vi "aquisicao.vi"() -> ()   [LabVIEW 2018]
uses:
  <vilib>/DAQmx/read.llb/DAQmx Read (Analog 1D Wfm NChan NSamp).vi
  <vilib>/DAQmx/create/channels.llb/DAQmx Create Channel (AI-Voltage-Basic).vi
  <vilib>/DAQmx/configure/timing.llb/DAQmx Timing (Sample Clock).vi
  <vilib>/DAQmx/miscellaneous.llb/DAQmx Fill In Error Info.vi
panel:
  in  "Parar":bool caption="stop"
  out "Onda Gerada":waveform(dbl)[](graph)
  # "Validação da Onda Gerada"
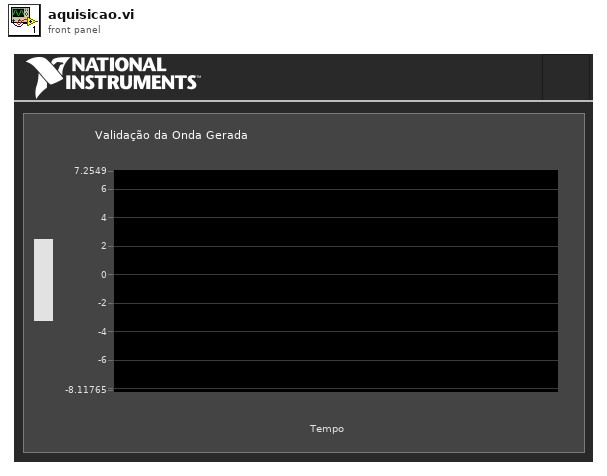
[diagram p1: front panel]
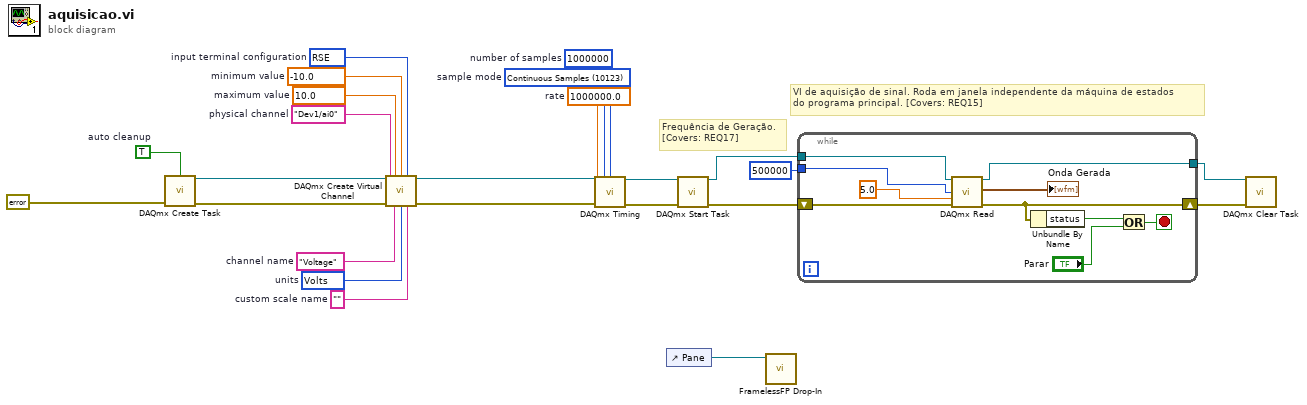
[diagram p0: block diagram]
diagram:
  w17 = 10123 items=["Finite Samples"=10178, "Continuous Samples"=10123, "Hardware Timed Single Point"=12522]  # sample mode
  w16 = 1000000  # number of samples
  w15 = 1000000.0  # rate
  w13 = 10083 items=["default"=-1, "RSE"=10083, "NRSE"=10078, "Differential"=10106, "Pseudodifferential"=12529]  # input terminal configuration
  w12 = 10348 items=["Volts"=10348, "From Custom Scale"=10065]  # units
  w11 = "Voltage"  # channel name
  w9 = ""  # custom scale name
  w8 = -10.0  # minimum value
  w7 = 10.0  # maximum value
  w6 = "Dev1/ai0"  # physical channel
  w4 = TRUE  # auto cleanup
  # "Frequência de Geração.\n[Covers: REQ17]"
  # "VI de aquisição de sinal. Roda em janela independente da máquina de estados\ndo programa principal. [Covers: REQ15]"
  n1 = call <vilib>:"DAQmx Create Task.vi"("auto cleanup"=w4, "error in"=errorcluster {"status"=FALSE, "code"=0, "source"=""}) -> ("task out"=w5:refnum<k21>, "error out"=w3:errorcluster)  [unwired: 12 in]
  n2 = call-poly <vilib>:"DAQmx Create Virtual Channel.vi"("task in"=w5, "maximum value"=w7, "minimum value"=w8, "input terminal configuration"=w13, "physical channels"=w6, "name to assign"=w11, "units"=w12, "error in"=w3, "custom scale name"=w9) -> ("task out"=w14:refnum<k21>, "error out"=w10:errorcluster)  [unwired: 5 in]
  n3 = call-poly <vilib>:"DAQmx Timing.vi"("task/channels in"=w14, "sample mode"=w17, "samples per channel"=w16, "rate"=w15, "error in"=w10) -> ("task out"=w19:refnum<k21>, "error out"=w18:errorcluster)  [unwired: 9 in]
  n4 = control-ref of="Pane"() -> (w2:refnum<vi>)
  n5 = call <vilib>:"DAQmx Start Task.vi"("task/channels in"=w19, "error in"=w18) -> ("task out"=w24:refnum<k21>, "error out"=w23:errorcluster)  [unwired: 12 in]
  n6 = call "FramelessFP Drop-In.vi"("Pane in"=w2) -> ()  [unwired: 10 in, 1 out]
  n7 = while {
    tunnel: w24 -> [w34]
    tunnel: 500000 ("number of samples") -> [w31]
    tunnel: [w32] -> w20
    shift-right: [w29] -> w21
    shift-left: w23 -> [w33]
    stop <- w28 stop-if-true
    n8 = call-poly <vilib>:"DAQmx Read.vi"("task/channels in"=w34, "number of samples per channel"=w31, "timeout"=5.0 ("timeout (s)"), "error in"=w33) -> ("task out"=w32:refnum<k21>, "data"=→"Onda Gerada":waveform(dbl)[], "error out"=w29:errorcluster)  [unwired: 9 in]
    n9 = Unbundle By Name(w29) -> ("status"=w30:bool)
    n10 = Or(x=w30, y="Parar") -> (x .or. y?=w28:bool)
  }
  n11 = call <vilib>:"DAQmx Clear Task.vi"("task in"=w20, "error in"=w21) -> ()  [unwired: 13 in, 1 out]
